vi "Pre-Create Glimpse File.vi"(3 "pre-created file #":u16=10, 4 "Select a Folder":path) -> (0 "Path Array":path[](array[path]), 1 "refnum Array":refnum<file>[](array[refnum]), 2 "Path String Array":string[](array[string]))   [LabVIEW 2014]
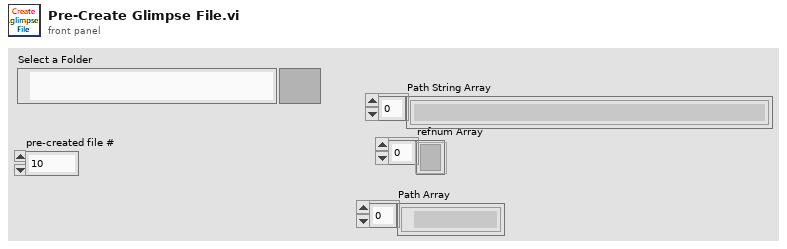
[diagram p1: front panel]
types:
  T1 = enum16{"open", "replace", "create", "open or create", "replace or create", "replace or create with confirmation"}
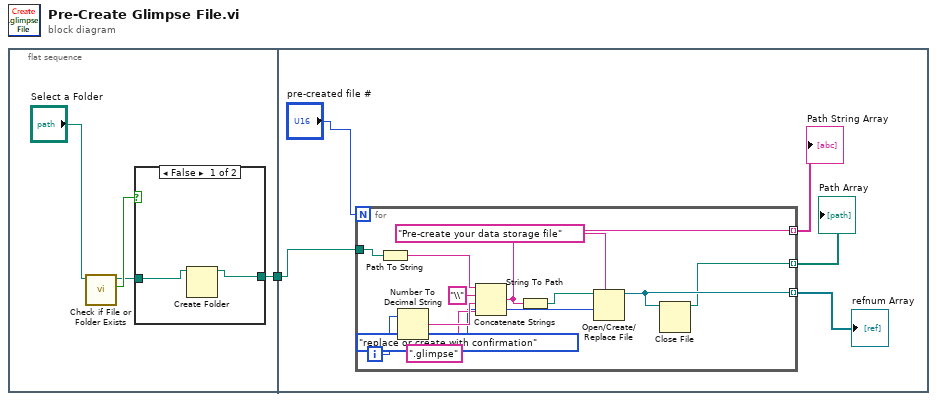
[diagram p0: block diagram]
diagram:
  n1 = flat-sequence {
    tunnel: [w2] -> w1
    tunnel: w1 -> [w11]
    frame #0 {
      n2 = call <vilib>:"Check if File or Folder Exists.vi"("path"="Select a Folder") -> ("file or folder exists?"=w4:bool, "dup path"=w3:path)  [unwired: 8 in, 1 out]
      n3 = case shown="False" w4 {
        tunnel: [w6 w8] -> w2
        tunnel: w3 -> [w7 w8]
        frame False {
          n4 = Create Folder(path (use dialog)=w7) -> (created path=w6:path)  [unwired: 2 in, 2 out]
        }
        frame True {
        }
      }
    }
    frame #1 {
      n5 = for {
        N: "pre-created file #" -> [_]
        tunnel: w11 -> [w25]
        tunnel: [w15] -> w12 mode=indexing
        tunnel: [w18] -> w13 mode=indexing
        tunnel: [w14] -> w9 mode=indexing
        i -> [w24]
        n6 = Path To String(path=w25) -> (string=w20:string)
        n7 = Number To Decimal String(number=w24) -> (decimal integer string=w23:string)  [unwired: 1 in]
        n8 = Concatenate Strings(w20, "\\" ("string"), w23, ".glimpse" ("string")) -> (w18:string)
        n9 = String To Path(string=w18) -> (path=w16:path)
        n10 = Open/Create/Replace File(file path (use dialog)=w16, prompt="Pre-create your data storage file", operation (0:open)=T1."replace or create with confirmation") -> (refnum out=w15:refnum<file>)  [unwired: 3 in, 2 out]
        n11 = Close File(refnum=w15) -> (path=w14:path)  [unwired: 1 in, 1 out]
      }
      "refnum Array" <- w12
      "Path String Array" <- w13
      "Path Array" <- w9
    }
  }
